vi "SET_PWM.vi"(8 "error in (no error)":errorcluster, 9 "PWM":dbl, 10 "STATE":T1(ring), 11 "Serial Data Gcode":refnum<queue>) -> (0 "error out":errorcluster)   [LabVIEW 2017]
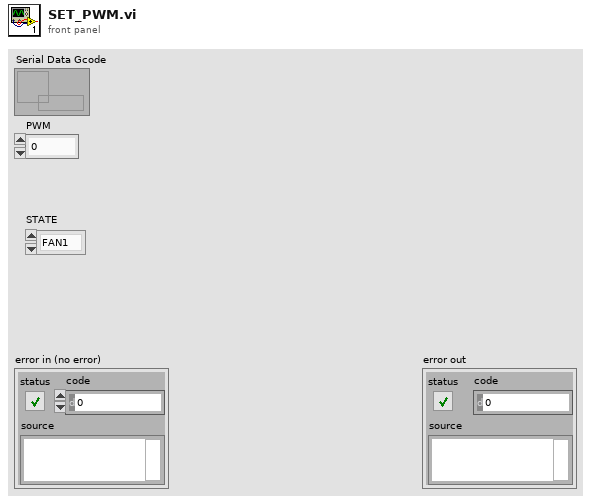
[diagram p1: front panel]
types:
  T1 = enum16{"FAN1", "FAN2", "FAN3", "SPINDLE", "LASER", "SOLENOID"}
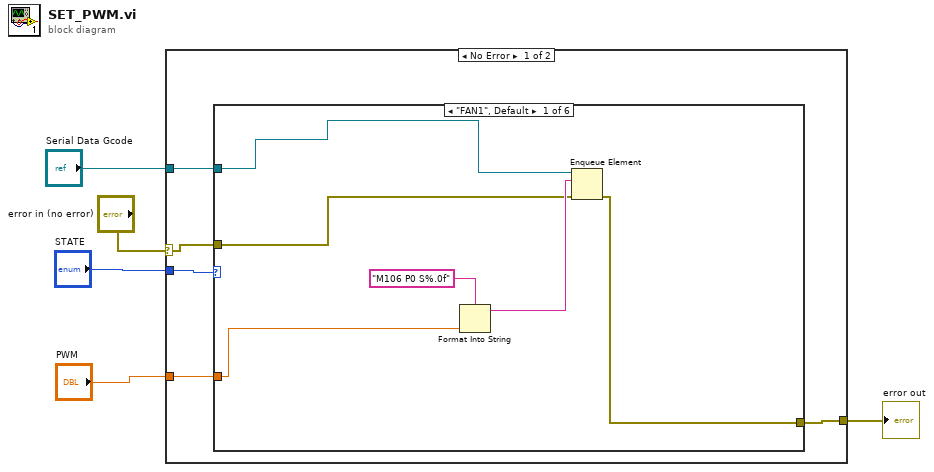
[diagram p0: block diagram]
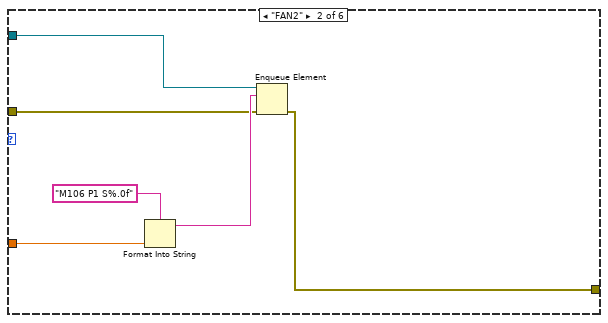
[diagram p2: hidden frame]
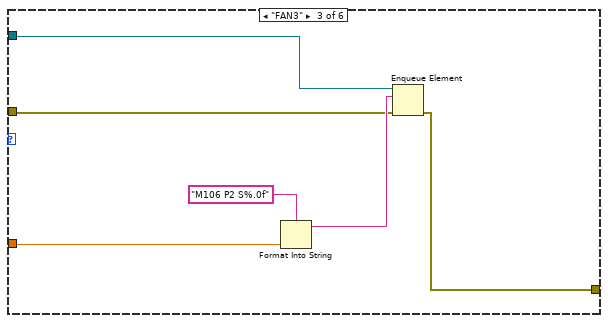
[diagram p3: hidden frame]
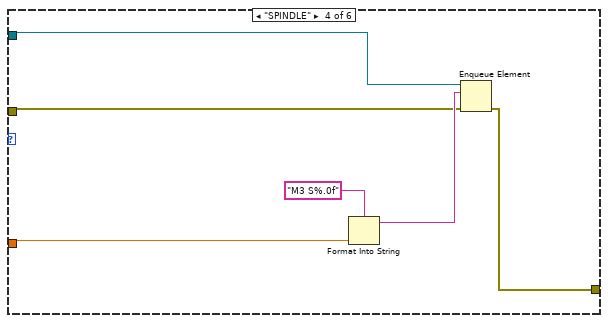
[diagram p4: hidden frame]
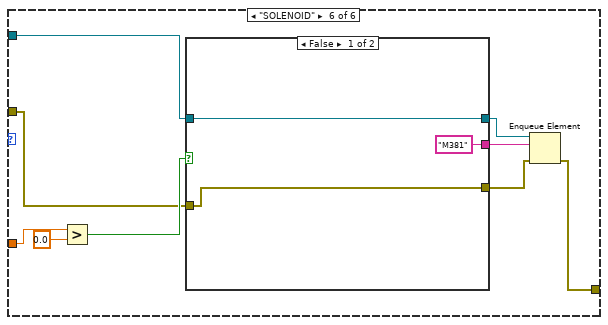
[diagram p6: hidden frame]
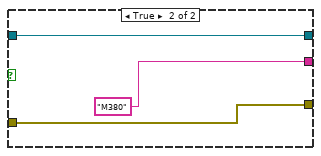
[diagram p7: hidden frame]
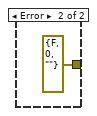
[diagram p8: hidden frame]
diagram:
  n1 = case shown="No Error" "error in (no error)" {
    selector: "error in (no error)" -> [w8 _]
    tunnel: "STATE" -> [w10 _]
    tunnel: [w9 errorcluster {"status"=FALSE, "code"=0, "source"=""} ("error out")] -> w4
    tunnel: "Serial Data Gcode" -> [w7 _]
    tunnel: "PWM" -> [w6 _]
    frame No Error {
      n2 = case shown="\"FAN1\", Default" w10 {
        tunnel: [w11 w20 w26 w29 w35 w36] -> w9
        tunnel: w8 -> [w13 w19 w24 w31 w35 w38]
        tunnel: w7 -> [w14 w18 w25 w32 _ w41]
        tunnel: w6 -> [w12 w17 w23 w30 _ w44]
        frame "FAN1", Default {
          n3 = Format Into String(format string="M106 P0 S%.0f", w12) -> (resulting string=w15:string)  [unwired: 2 in, 1 out]
          n4 = Enqueue Element(queue=w14, element=w15, error in (no error)=w13) -> (error out=w11:errorcluster)  [unwired: 1 in, 2 out]
        }
        frame "FAN2" {
          n5 = Format Into String(format string="M106 P1 S%.0f", w17) -> (resulting string=w21:string)  [unwired: 2 in, 1 out]
          n6 = Enqueue Element(queue=w18, element=w21, error in (no error)=w19) -> (error out=w20:errorcluster)  [unwired: 1 in, 2 out]
        }
        frame "FAN3" {
          n7 = Format Into String(format string="M106 P2 S%.0f", w23) -> (resulting string=w27:string)  [unwired: 2 in, 1 out]
          n8 = Enqueue Element(queue=w25, element=w27, error in (no error)=w24) -> (error out=w26:errorcluster)  [unwired: 1 in, 2 out]
        }
        frame "SPINDLE" {
          n9 = Format Into String(format string="M3 S%.0f", w30) -> (resulting string=w33:string)  [unwired: 2 in, 1 out]
          n10 = Enqueue Element(queue=w32, element=w33, error in (no error)=w31) -> (error out=w29:errorcluster)  [unwired: 1 in, 2 out]
        }
        frame "LASER" {
        }
        frame "SOLENOID" {
          n11 = Greater?(x=w44, y=0.0) -> (0:w42:bool)
          n12 = case shown="False" w42 {
            tunnel: w41 -> [w46 w49]
            tunnel: w38 -> [w45 w48]
            tunnel: ["M381" ("element") "M380" ("element")] -> w40
            tunnel: [w46 w49] -> w39
            tunnel: [w45 w48] -> w37
            frame False {
            }
            frame True {
            }
          }
          n13 = Enqueue Element(queue=w39, element=w40, error in (no error)=w37) -> (error out=w36:errorcluster)  [unwired: 1 in, 2 out]
        }
      }
    }
    frame Error {
    }
  }
  "error out" <- w4
